vi "Round.vi"() -> (3 "Round":i32)   [LabVIEW 2020, in "Square.lvclass"]
uses:
  Square.lvclass
  SubVIs/Globals (private).vi
  SubVIs/SB SubVIs.lvlib
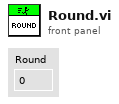
[diagram p1: front panel]
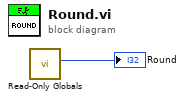
[diagram p0: block diagram]
diagram:
  n1 = call "Read-Only Globals.vi"() -> ("Round"=→"Round":i32)  [unwired: 10 in, 1 out]
